vi "Com_Find Ports.vi"() -> (2 "Com Numbers":i32[](array[numeric]), 3 "Com array":string[](array[string]))   [LabVIEW 2020]
uses:
  <vilib>/Instr/_visa.llb/VISA Find Search Mode.ctl
panel:
  out "find list":string[](array[string])
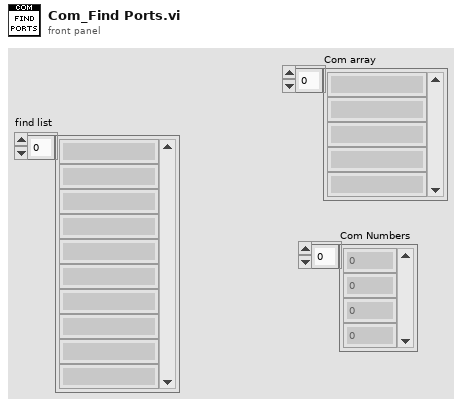
[diagram p1: front panel]
types:
  T1 = typedef "VISA Find Search Mode.ctl" = u32
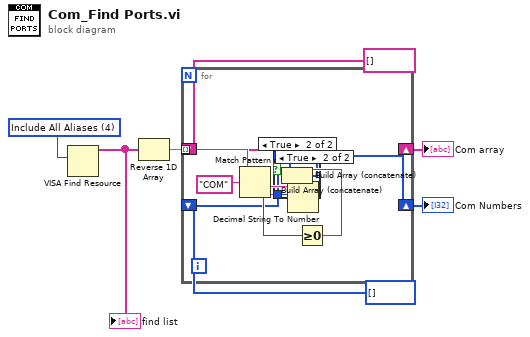
[diagram p0: block diagram]
diagram:
  w7 = T1 4 items=["Canonical Names Only"=0, "Aliases Only"=2, "Include Matching Aliases"=3, "Include All Aliases"=4] ("Search Mode")
  n1 = VISA Find Resource(10:w7) -> (3:w6:string[])  [unwired: 2 in, 2 out]
  "find list" <- w6
  n2 = Reverse 1D Array(array=w6) -> (reversed array=w3:string[])
  n3 = for {
    tunnel: w3 -> [w13] mode=indexing
    shift-right: [w10] -> w4
    shift-left: i32[] [] ("Array") -> [w11]
    shift-right: [w8] -> w5
    shift-left: string[] [] ("Array") -> [w9]
    n4 = Match Pattern(string=w13, regular expression="COM") -> (after substring=w12:string, offset past match=w15:i32)  [unwired: 1 in, 2 out]
    n5 = Decimal String To Number(string=w12) -> (number=w16:i32)  [unwired: 2 in, 1 out]
    n6 = Greater Or Equal To 0?(x=w15) -> (x >= 0?=w14:bool)
    n7 = case shown="True" w14 {
      tunnel: w9 -> [w18 w20]
      tunnel: w13 -> [_ w19]
      tunnel: [w18 w21] -> w8
      frame False {
      }
      frame True {
        n8 = Build Array (concatenate)(w20, w19) -> (w21:string[])
      }
    }
    n9 = case shown="True" w14 {
      tunnel: w11 -> [w22 w24]
      tunnel: w16 -> [_ w23]
      tunnel: [w22 w25] -> w10
      frame False {
      }
      frame True {
        n10 = Build Array (concatenate)(w24, w23) -> (w25:i32[])
      }
    }
  }
  "Com array" <- w5
  "Com Numbers" <- w4
